vi "Drive Check for New Command.vi"(9 "input cluster":T7, 10 "Wait time (ms)":dbl, 11 "Finished?":bool) -> (0 "Completion":T4, 1 "Subsystem Name":string, 2 "Current Command":T1, 3 "Initial Trace String":string, 4 "Next Command":T6)   [LabVIEW 2023]
doc: "This VI is called for each controller loop iteration. It checks for new commands, updates timing data, and upon completion, notifies and waiting commands."
uses:
  Drive Setpoints.ctl
  Drive Operations.ctl
  <vilib>/Rock Robotics/WPI/Framework/Command Status Info.ctl
  <vilib>/Rock Robotics/WPI/Framework/Completion Status.ctl
  <vilib>/Rock Robotics/WPI/Framework/Completion Notifier.ctl
  Drive Published Globals.vi
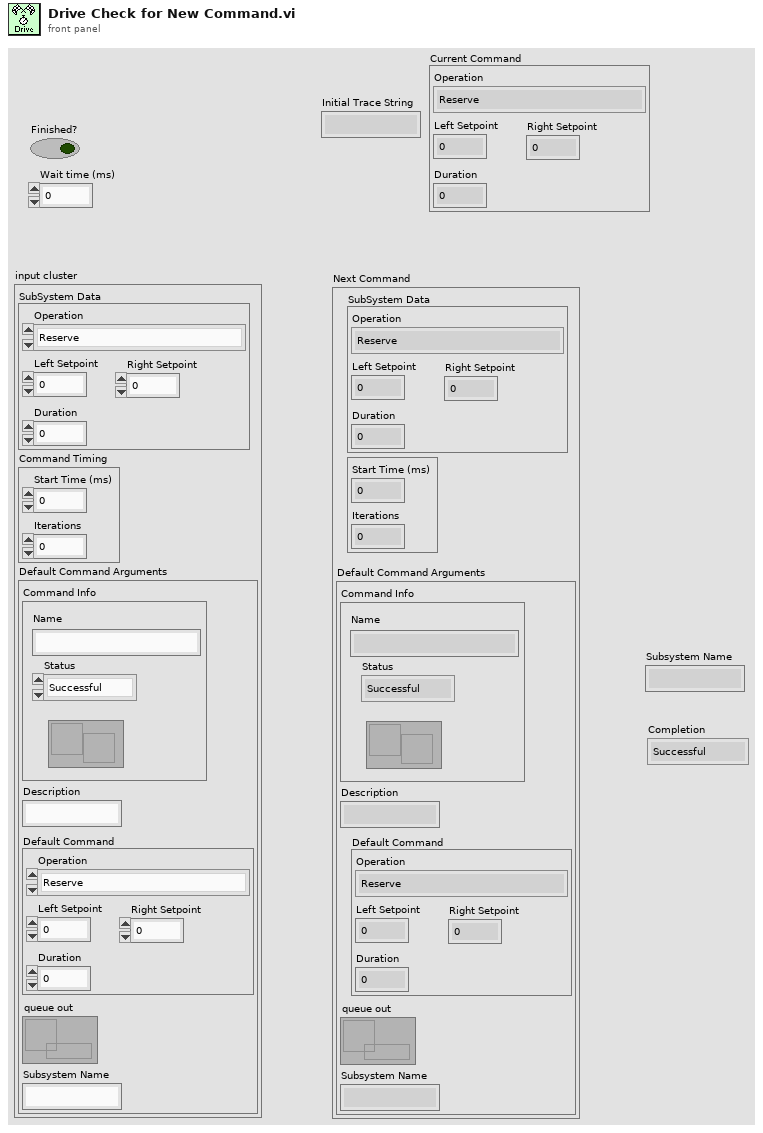
[diagram p1: front panel]
types:
  T1 = typedef "Drive Setpoints.ctl" = cluster{"Operation":T2, "Left Setpoint":dbl, "Right Setpoint":dbl, "Duration":dbl}
  T2 = typedef "Drive Operations.ctl" = enum16{"Reserve", "Read Current", "Immediate", "Drive for Time", "Drive for Distance"}
  T3 = typedef "Command Status Info.ctl" = cluster{"Name":string, "Status":T4, "notifier out":T5}
  T4 = typedef "Completion Status.ctl" = enum16{"Successful", "Aborted", "Incomplete"}
  T5 = typedef "Completion Notifier.ctl" = refnum<notifier>
  T6 = cluster{"SubSystem Data":T1, cluster{"Start Time (ms)":u32, "Iterations":i32}, "Default Command Arguments":cluster{"Command Info":T3, "Description":string, "Default Command":T1, "queue out":refnum<queue>, "Subsystem Name":string}}
  T7 = cluster{"SubSystem Data":T1, "Command Timing":cluster{"Start Time (ms)":u32, "Iterations":i32}, "Default Command Arguments":cluster{"Command Info":T3, "Description":string, "Default Command":T1, "queue out":refnum<queue>, "Subsystem Name":string}}
  T8 = cluster{"Command Info":T3, "Description":string, "Default Command":T1, "queue out":refnum<queue>, "Subsystem Name":string}
  T9 = cluster{"Default Command":T1, "Command Info":T3, "Description":string}
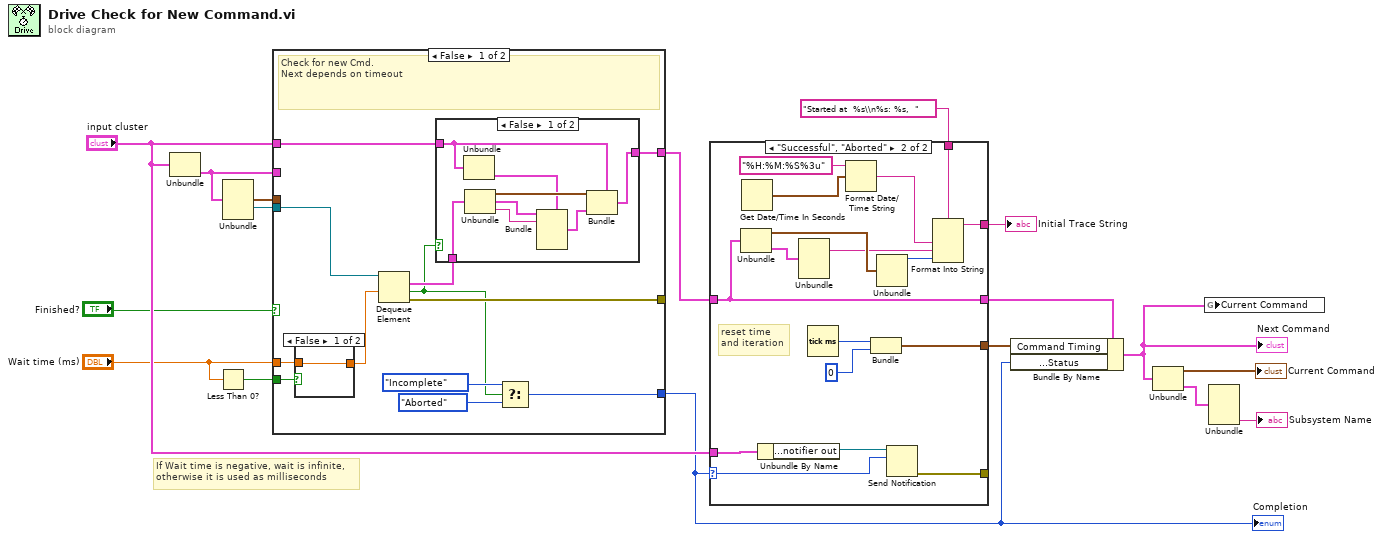
[diagram p0: block diagram]
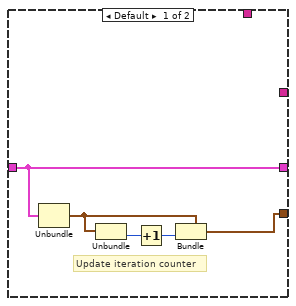
[diagram p2: hidden frame]
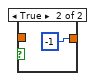
[diagram p4: hidden frame]
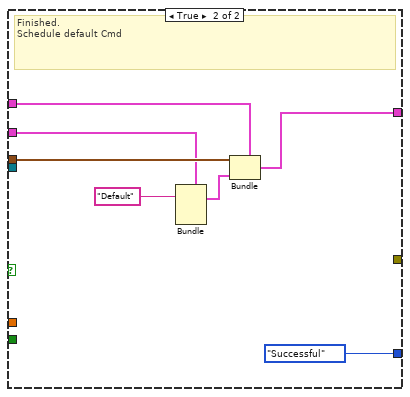
[diagram p5: hidden frame]
diagram:
  # "If Wait time is negative, wait is infinite,\notherwise it is used as milliseconds"
  n1 = Unbundle("input cluster") -> ("Default Command Arguments"=w7:T8)  [unwired: 2 out]
  n2 = Less Than 0?(x="Wait time (ms)") -> (x < 0?=w6:bool)
  n3 = Unbundle(w7) -> ("Default Command"=w10:T1, "queue out"=w11:refnum<queue>)  [unwired: 3 out]
  n4 = case shown="False" "Finished?" {
    tunnel: [w25 w46] -> w14
    tunnel: w6 -> [w19 _]
    tunnel: [w29 Completion_Status."Successful"] -> w1
    tunnel: [w22 _] -> _
    tunnel: w11 -> [w24 _]
    tunnel: "input cluster" -> [w26 w45]
    tunnel: w10 -> [_ w44]
    tunnel: w7 -> [_ w42]
    tunnel: "Wait time (ms)" -> [w18 _]
    frame False {
      # "Check for new Cmd.\nNext depends on timeout"
      n5 = case shown="False" w19 {
        tunnel: [w39 -1] -> w23
        tunnel: w18 -> [w39 _]
        frame False {
        }
        frame True {
        }
      }
      n6 = Dequeue Element(queue=w24, timeout in ms (-1)=w23) -> (element=w21:T9, timed out?=w20:bool, error out=w22:errorcluster)  [unwired: 1 in, 1 out]
      n7 = case shown="False" w20 {
        tunnel: w21 -> [w37 _]
        tunnel: w26 -> [w34 w38]
        tunnel: [w30 w38] -> w25
        frame False {
          n8 = Unbundle(w34) -> ("Default Command Arguments"=w33:T8)  [unwired: 2 out]
          n9 = Unbundle(w37) -> ("Default Command"=w36:T1, "Command Info"=w31:T3, "Description"=w32:string)
          n10 = Bundle(cluster=w33, "Command Info"=w31, "Description"=w32) -> (w35:T8)  [unwired: 3 in]
          n11 = Bundle(cluster=w34, "SubSystem Data"=w36, "Default Command Arguments"=w35) -> (w30:T7)  [unwired: 1 in]
        }
        frame True {
        }
      }
      n12 = Select(t=Completion_Status."Incomplete", s=w20, f=Completion_Status."Aborted") -> (s? t:f=w29:T4)
    }
    frame True {
      # "Finished.\nSchedule default Cmd"
      n13 = Bundle(cluster=w42, "Description"="Default") -> (w43:T8)  [unwired: 4 in]
      n14 = Bundle(cluster=w45, "SubSystem Data"=w44, "Default Command Arguments"=w43) -> (w46:T7)  [unwired: 1 in]
    }
  }
  "Completion" <- w1
  n15 = case shown="\"Successful\", \"Aborted\"" w1 {
    selector: w1 -> [_ w69]
    tunnel: "input cluster" -> [_ w60]
    tunnel: "Started at  %s\\n%s: %s,  " ("format string") -> [_ w66]
    tunnel: [_ w65] -> w16
    tunnel: w14 -> [w48 w53]
    tunnel: [w49 w54] -> w3
    tunnel: [_ w61] -> _
    tunnel: [w48 w53] -> w4
    frame Default {
      # "Update iteration counter"
      n16 = Unbundle(w48) -> ("Command Timing"=w50:cluster{"Start Time (ms)":u32, "Iterations":i32})  [unwired: 2 out]
      n17 = Unbundle(w50) -> ("Iterations"=w51:i32)  [unwired: 1 out]
      n18 = Increment(x=w51) -> (x+1=w52:i32)
      n19 = Bundle(cluster=w50, "Iterations"=w52) -> (w49:cluster{"Start Time (ms)":u32, "Iterations":i32})  [unwired: 1 in]
    }
    frame "Successful", "Aborted" {
      # "reset time\nand iteration"
      n20 = Unbundle(w53) -> ("SubSystem Data"=w64:T1, "Default Command Arguments"=w62:T8)  [unwired: 1 out]
      n21 = Get Date/Time In Seconds() -> (seconds since 1Jan1904=w56:timestamp)
      n22 = Unbundle By Name(w60) -> ("Default Command Arguments.Command Info.notifier out"=w68:T5)
      n23 = Unbundle(w62) -> ("Description"=w58:string)  [unwired: 4 out]
      n24 = Tick Count (ms)() -> (millisecond timer value=w59:u32)
      n25 = Format Date/Time String(time format string (%c)="%H:%M:%S%3u", seconds (now)=w56) -> (date/time string=w55:string)  [unwired: 1 in]
      n26 = Bundle("millisecond timer value"=w59, 0) -> (w54:cluster{"millisecond timer value":u32, i32})  [unwired: 1 in]
      n27 = Unbundle(w64) -> ("Operation"=w67:T2)  [unwired: 3 out]
      n28 = Send Notification(notification=w69, notifier=w68) -> (error out=w61:errorcluster)  [unwired: 1 in, 1 out]
      n29 = Format Into String(format string=w66, w55, w58, w67) -> (resulting string=w65:string)  [unwired: 2 in, 1 out]
    }
  }
  "Initial Trace String" <- w16
  n30 = Bundle By Name(cluster=w4, "Command Timing"=w3, "Default Command Arguments.Command Info.Status"=w1) -> (w2:T7)
  "Next Command" <- w2
  n31 = Unbundle(w2) -> ("SubSystem Data"=→"Current Command":T1, "Default Command Arguments"=w9:T8)  [unwired: 1 out]
  n32 = global write "Drive Published Globals.vi" "Current Command"(w2) -> ()
  n33 = Unbundle(w9) -> ("Subsystem Name"=→"Subsystem Name":string)  [unwired: 4 out]
